vi "Init Options.vi"(8 "error in (no error)":errorcluster {"code" format="%.0x"}, 11 "VISA Resource Name":refnum<visa-resource-name>) -> (0 "error out":errorcluster {"code" format="%.0x"}, 3 "VISA Resource Name Out":refnum<visa-resource-name>)   [LabVIEW 2011, in "Agilent 546XX Series.lvlib"]
doc: "This VI aborts an acquisition and returns the oscilloscope to the Idle state. You initiate an acquisition with the tktds3k Read Waveform, tktds3k Read Min Max Waveform, tktds3k Read Waveform Measurement, and tktds3k Initiate Acquisition VIs.\n\nNotes:\n\n(1) This VI does not check the instrument status. Typically, you call this VI only in a sequence of calls to other low-level driver VIs. The sequence performs one operation. You use the low-level VIs to optimize one or more aspects of interaction with the instrument. If you want to check the instrument status, call the tktds3k Error-Query VI at the conclusion of the sequence."
uses:
  Agilent 546XX Series.lvlib
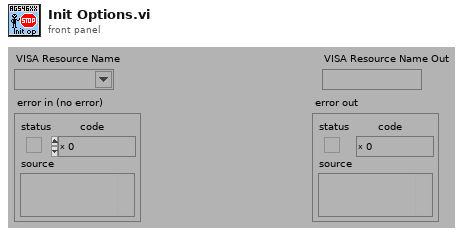
[diagram p1: front panel]
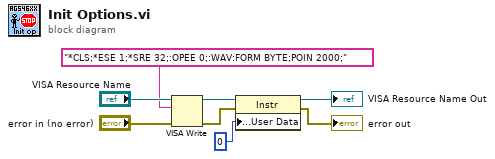
[diagram p0: block diagram]
diagram:
  n1 = VISA Write(VISA resource name="VISA Resource Name", write buffer="*CLS;*ESE 1;*SRE 32;:OPEE 0;:WAV:FORM BYTE;POIN 2000;", error in (no error)="error in (no error)") -> (VISA resource name out=w4:refnum<visa-resource-name>, error out=w2:errorcluster)  [unwired: 1 out]
  n2 = property class="Instr"(reference=w4, error in=w2, "General Settings:User Data"=u32 0) -> (reference out=→"VISA Resource Name Out":refnum<visa-resource-name>, error out=→"error out":errorcluster)
